vi "AnimatorFacade.vi"(0 "Data In":T6, 2 "Display State In":T2, 3 "Container State":T5) -> (6 "Data Out":T6, 7 "Display State Out":T2, 8 "Action":T1)   [LabVIEW 2019, in "AnimatorXControl.xctl"]
uses:
  AnimatorXControl.xctl
  AnimatorData.ctl
  <vilib>/_xctls/Container State.ctl
  AnimatorState.ctl
  <vilib>/picture/picture.llb/imagedata.ctl
  AnimatorSettings.ctl
  <vilib>/_xctls/Action.ctl
  AnimatorCommand.ctl
  <vilib>/_xctls/XControlSupport.lvlib
panel:
  out "Picture":picture
types:
  T1 = typedef "XControlSupport.lvlib/Action.ctl" = cluster{"Data Changed?":bool, "State Changed?":bool, "Action Name":string}
  T2 = typedef "AnimatorXControl.xctl/AnimatorState.ctl" = cluster{"Images":cluster{"Files":path[], "ImageData":T3[]}, "Settings":T4}
  T3 = typedef "imagedata.ctl" = cluster{"image type":i32, "image depth":i32, "image":u8[], "mask":u8[], "colors":u32[], "Rectangle":cluster{"left":i16, "top":i16, "right":i16, "bottom":i16}}
  T4 = typedef "AnimatorXControl.xctl/AnimatorSettings.ctl" = cluster{"Reverse":bool, "FrameRate":dbl, "WorkMode":enum16{"Automatic", "UseValue"}}
  T5 = typedef "XControlSupport.lvlib/Container State.ctl" = cluster{"Indicator?":bool, "Run Mode?":bool, " Refnum":refnum<vi>}
  T6 = typedef "AnimatorXControl.xctl/AnimatorData.ctl" = u32
  T7 = typedef "AnimatorXControl.xctl/AnimatorCommand.ctl" = enum16{"AddAnimator", "RemoveAnimator", "Settings"}
  T8 = cluster{"ImageData":picture[], "Pict Refnum":refnum<vi>}
  T9 = typedef "LVRectTypeDef.ctl" = cluster{"Left":i16, "Top":i16, "Right":i16, "Bottom":i16}
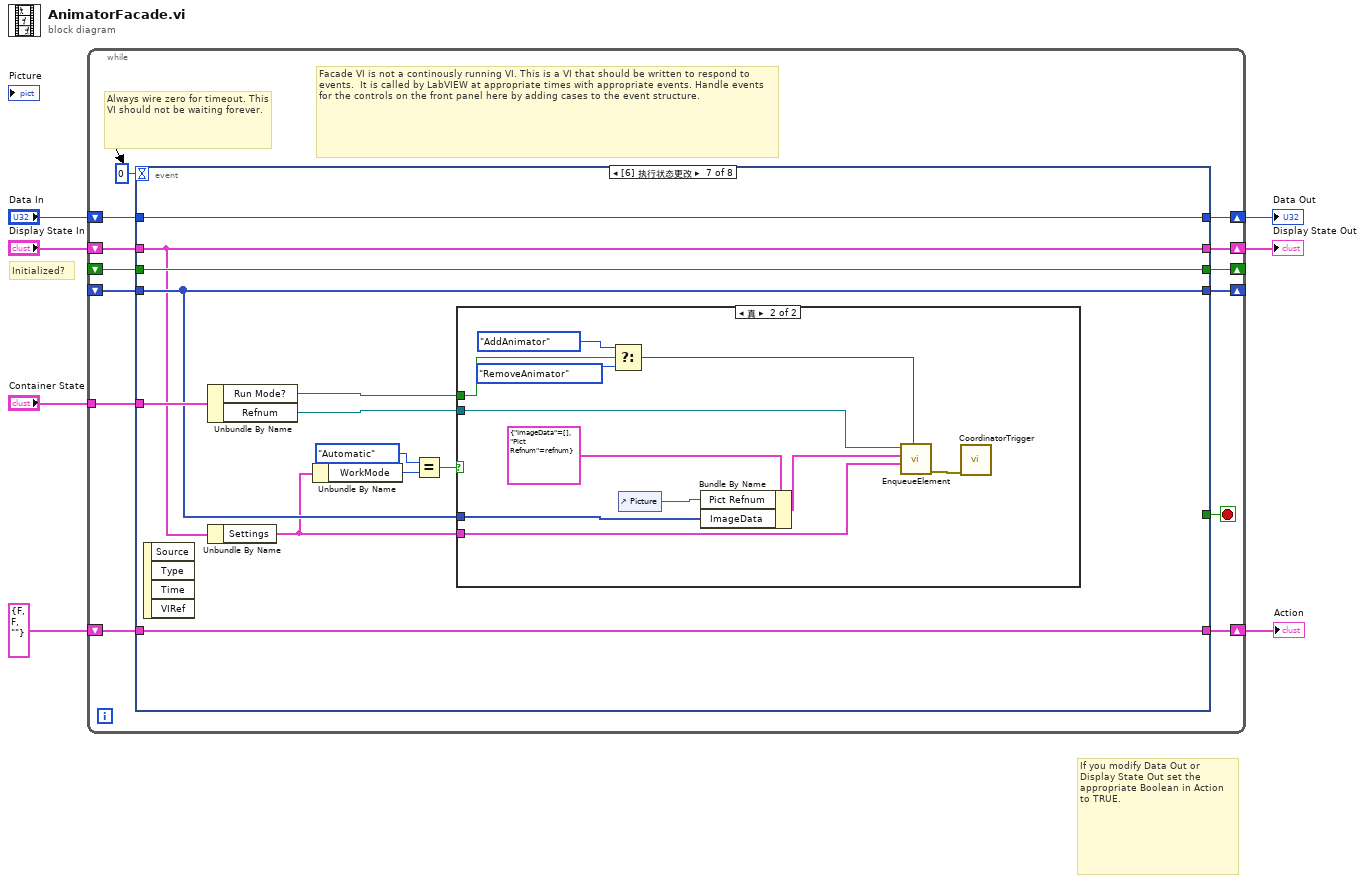
[diagram p0: block diagram]
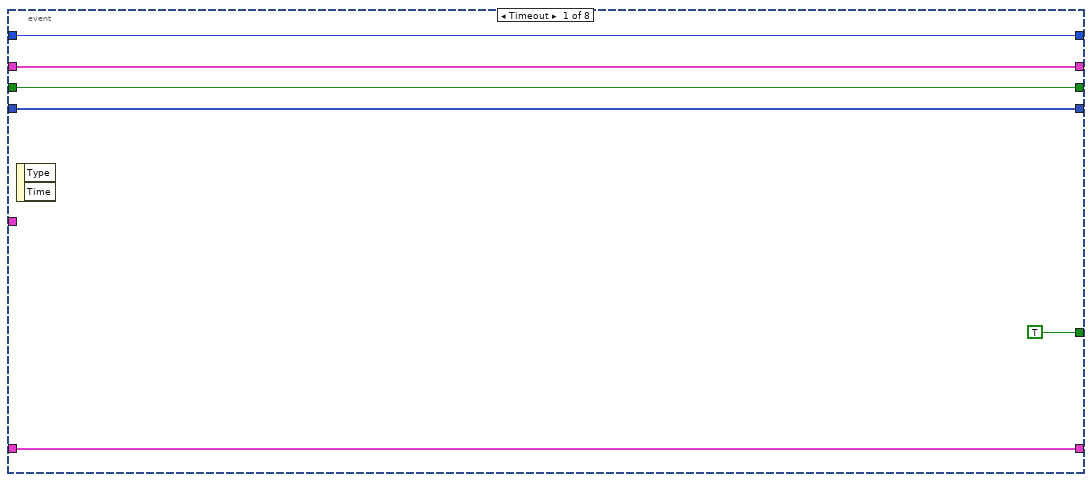
[diagram p2: hidden frame]
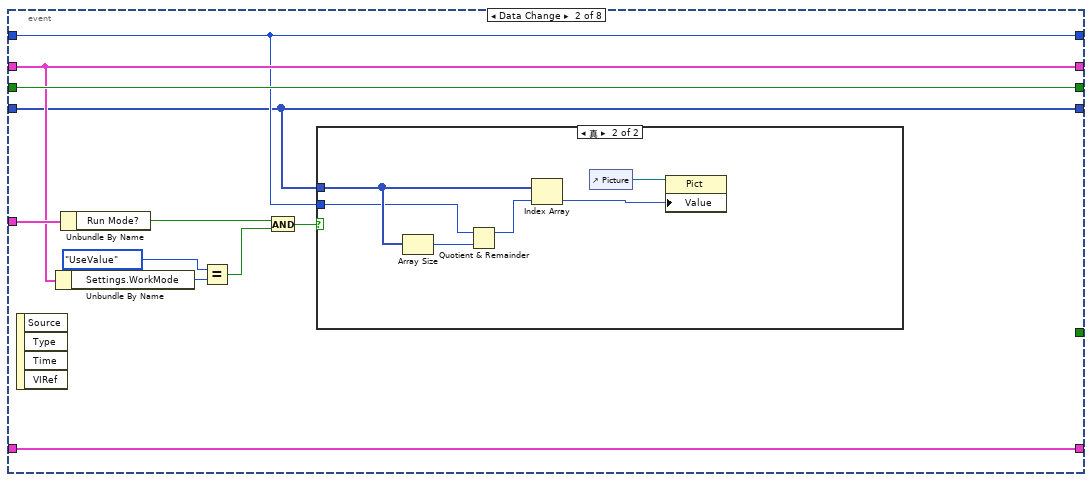
[diagram p3: hidden frame]
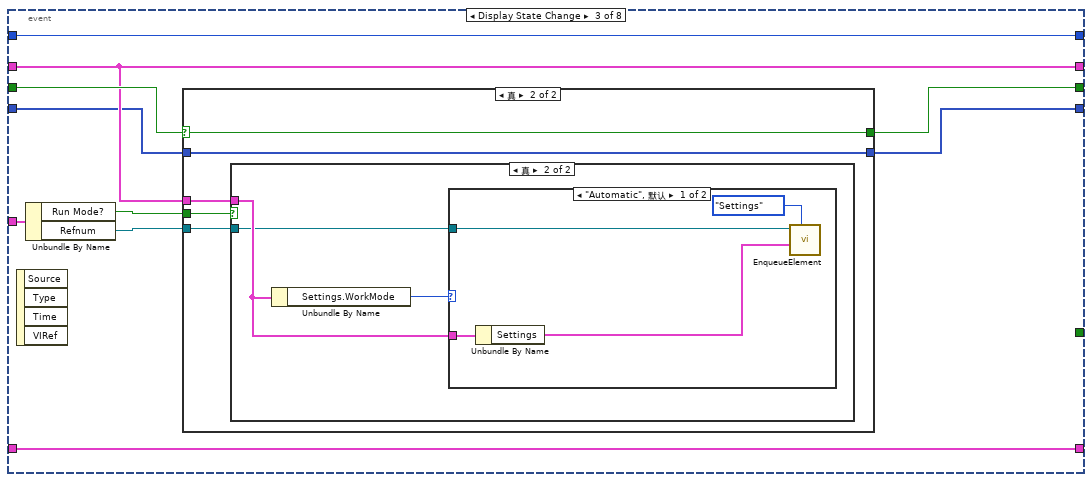
[diagram p5: hidden frame]
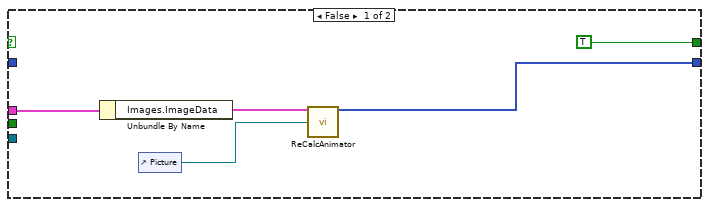
[diagram p6: hidden frame]
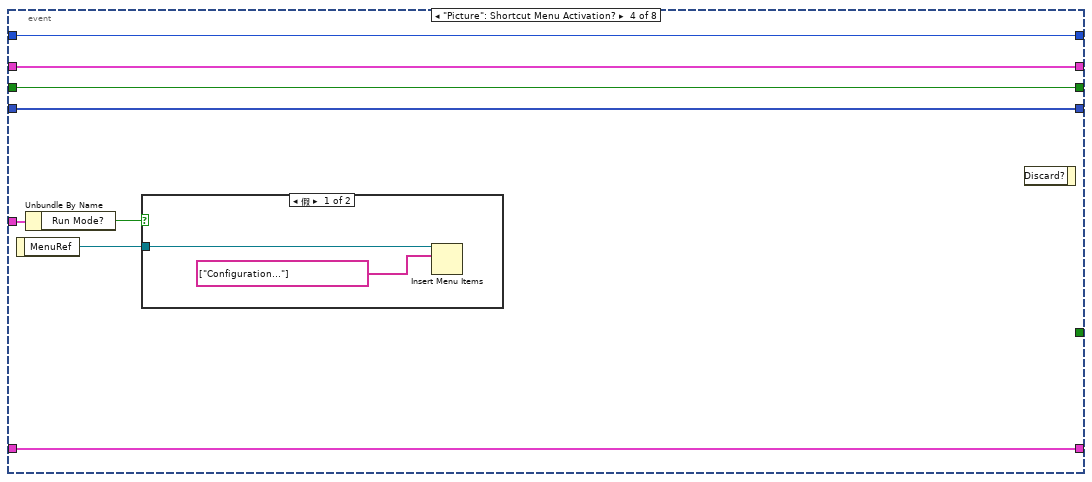
[diagram p9: hidden frame]
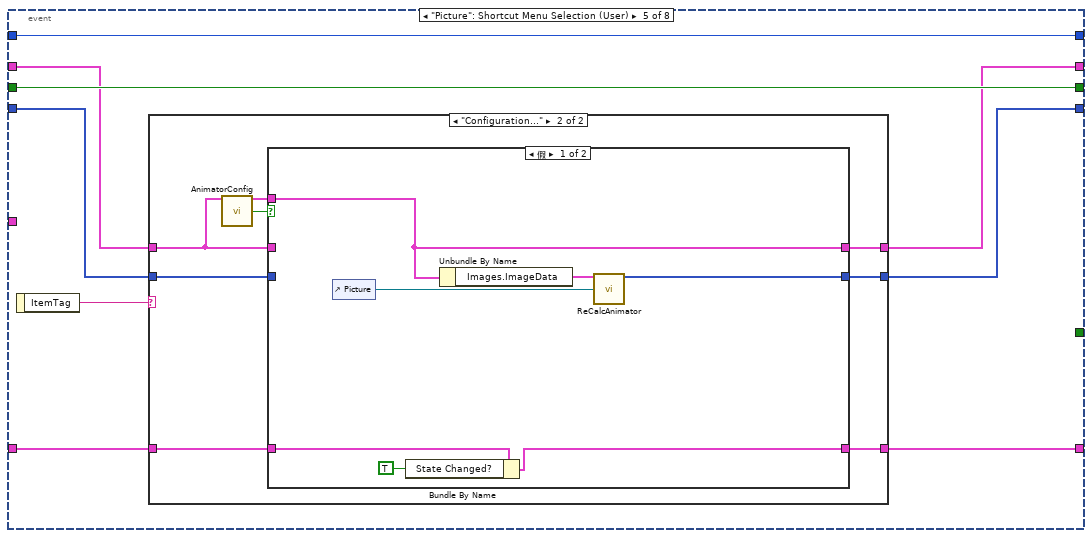
[diagram p11: hidden frame]
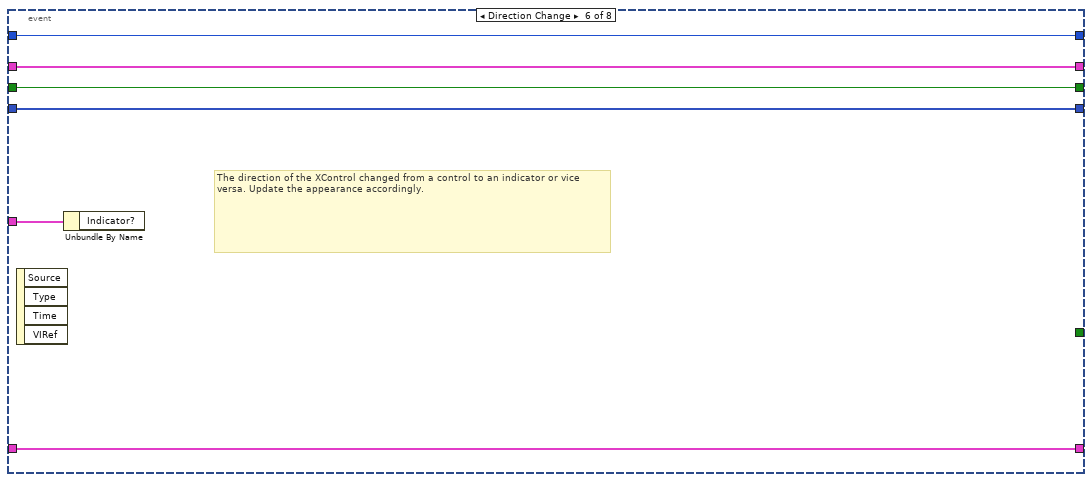
[diagram p14: hidden frame]
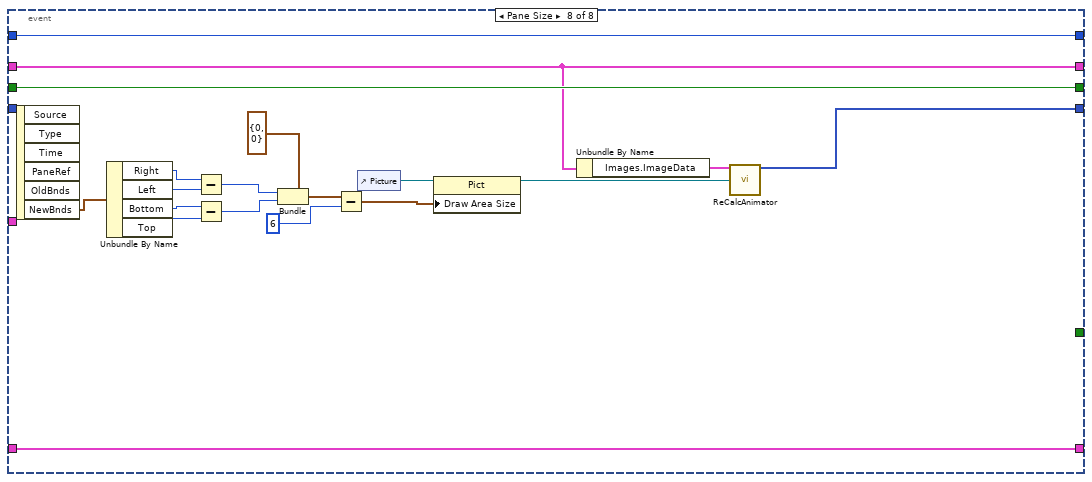
[diagram p16: hidden frame]
diagram:
  # "Initialized?"
  # "If you modify Data Out or\nDisplay State Out set the\nappropriate Boolean in Action\nto TRUE."
  n1 = while {
    shift-right: [w19] -> w4
    shift-left: "Display State In" -> [w20]
    tunnel: "Container State" -> [w16]
    shift-right: [w14] -> w7
    shift-left: "Data In" -> [w15]
    shift-right: [w12] -> w2
    shift-left: T1 {"Data Changed?"=FALSE, "State Changed?"=FALSE, "Action Name"=""} ("Action") -> [w13]
    shift-right: [w11] -> _
    shift-left: _ -> [w10]
    shift-right: [w8] -> _
    shift-left: _ -> [w9]
    stop <- w18 stop-if-true
    # "Facade VI is not a continously running VI. This is a VI that should be written to respond to events.  It is called by LabVIEW at appropriate times with appropriate events. Handle events for the controls on the front panel here by adding cases to the event structure."
    # "Always wire zero for timeout. This\nVI should not be waiting forever."
    n2 = event shown="[6] 执行状态更改" {
      selector: _ -> [_ _ _ _ _ _ _ _]
      dyn-events: _ -> [_ _ _ _ _ _ _ _]
      timeout: 0 -> [_ _ _ _ _ _ _ _]
      tunnel: w20 -> [w25 w34 w46 w74 w86 w115 w123 w144]
      tunnel: [w25 w34 w46 w74 w83 w115 w123 w144] -> w19
      tunnel: [TRUE _ _ _ _ _ _ _] -> w18
      tunnel: w16 -> [_ w35 w51 w78 _ w116 w128 _]
      tunnel: w15 -> [w24 w30 w53 w73 w89 w114 w127 w148]
      tunnel: [w24 w30 w53 w73 w89 w114 w127 w148] -> w14
      tunnel: [w26 w37 w47 w75 w84 w113 w126 w146] -> w12
      tunnel: w13 -> [w26 w37 w47 w75 w85 w113 w126 w146]
      tunnel: [w23 w36 w50 w72 w88 w112 w125 w147] -> w11
      tunnel: w10 -> [w23 w36 w52 w72 w88 w112 w125 w147]
      tunnel: w9 -> [w21 w29 w45 w71 w82 w111 w124 _]
      tunnel: [w21 w29 w44 w71 w81 w111 w124 w140] -> w8
      event Timeout {
        n3 = event-data() -> ()  [unwired: 1 in, 2 out]
      }
      event Data Change {
        n4 = event-data() -> ()  [unwired: 1 in, 4 out]
        n5 = Unbundle By Name(w34) -> ("Settings.WorkMode"=w32:enum16{"Automatic", "UseValue"})
        n6 = Unbundle By Name(w35) -> ("Run Mode?"=w28:bool)
        n7 = Equal?(x=enum16{"Automatic", "UseValue"}."UseValue", y=w32) -> (x = y?=w27:bool)
        n8 = And(x=w28, y=w27) -> (x .and. y?=w33:bool)
        n9 = case shown="真" w33 {
          tunnel: w30 -> [_ w38]
          tunnel: w29 -> [_ w43]
          frame False {
          }
          frame True {
            n10 = Array Size(array=w43) -> (size(s)=w39:i32)
            n11 = Quotient & Remainder(x=w38, y=w39) -> (x-y*floor(x/y)=w42:T6)  [unwired: 1 out]
            n12 = Index Array(array=w43, index=w42) -> (element=w40:picture)
            n13 = control-ref of="Picture"() -> (w41:refnum<vi>)
            n14 = property class="Pict"(reference=w41, "Value"=w40) -> ()  [unwired: 1 in, 2 out]
          }
        }
      }
      event Display State Change {
        n15 = event-data() -> ()  [unwired: 1 in, 4 out]
        n16 = Unbundle By Name(w51) -> ("Run Mode?"=w49:bool, "Refnum"=w48:refnum<vi>)
        n17 = case shown="真" w52 {
          selector: w52 -> [_ w63]
          tunnel: [TRUE w63] -> w50
          tunnel: w46 -> [w57 w61]
          tunnel: w49 -> [_ w62]
          tunnel: w48 -> [_ w60]
          tunnel: w45 -> [_ w59]
          tunnel: [w54 w59] -> w44
          frame False {
            n18 = Unbundle By Name(w57) -> ("Images.ImageData"=w55:T3[])
            n19 = control-ref of="Picture"() -> (w56:refnum<vi>)
            n20 = call "ReCalcAnimator.vi"("Image Array"=w55, "Pict Refnum"=w56) -> ("Pic Array"=w54:picture[])  [unwired: 12 in, 1 out]
          }
          frame True {
            n21 = case shown="真" w62 {
              tunnel: w61 -> [_ w65]
              tunnel: w60 -> [_ w64]
              frame False {
              }
              frame True {
                n22 = Unbundle By Name(w65) -> ("Settings.WorkMode"=w66:enum16{"Automatic", "UseValue"})
                n23 = case shown="\"Automatic\", 默认" w66 {
                  tunnel: w65 -> [w70 _]
                  tunnel: w64 -> [w68 _]
                  frame "Automatic", Default {
                    n24 = Unbundle By Name(w70) -> ("Settings"=w69:T4)
                    n25 = call "EnqueueElement.vi"("Command"=AnimatorCommand."Settings", "Settings"=w69, "XRefnum"=w68) -> ()  [unwired: 8 in, 1 out]
                  }
                  frame "UseValue" {
                  }
                }
              }
            }
          }
        }
      }
      event "Picture": Shortcut Menu Activation? {
        n26 = event-data() -> ("MenuRef"=w76:refnum<k9>)  [unwired: 1 in]
        n27 = Unbundle By Name(w78) -> ("Run Mode?"=w77:bool)
        n28 = case shown="假" w77 {
          tunnel: w76 -> [w80 _]
          frame False {
            n29 = Insert Menu Items(8:string[] ["Configuration..."] ("item names"), 9:w80) -> ()  [unwired: 4 in, 3 out]
          }
          frame True {
          }
        }
        n30 = event-data() -> ()  [unwired: 2 in, 1 out]
      }
      event "Picture": Shortcut Menu Selection (User) {
        n31 = event-data() -> ("ItemTag"=w87:string)  [unwired: 1 in]
        n32 = case shown="\"Configuration...\"" w87 {
          tunnel: w86 -> [w91 w96]
          tunnel: w85 -> [w92 w100]
          tunnel: [w92 w99] -> w84
          tunnel: [w91 w97] -> w83
          tunnel: [w90 w94] -> w81
          tunnel: w82 -> [w90 w93]
          frame Default {
          }
          frame "Configuration..." {
            n33 = call "AnimatorConfig.vi"("State In"=w96) -> ("State Out"=w98:T2, "Cancel?"=w95:bool)  [unwired: 12 in, 1 out]
            n34 = case shown="假" w95 {
              tunnel: w100 -> [w107 w110]
              tunnel: [w105 w110] -> w99
              tunnel: w98 -> [w104 _]
              tunnel: [w104 w109] -> w97
              tunnel: w96 -> [_ w109]
              tunnel: [w101 w108] -> w94
              tunnel: w93 -> [_ w108]
              frame False {
                n35 = control-ref of="Picture"() -> (w102:refnum<vi>)
                n36 = Bundle By Name(cluster=w107, "State Changed?"=TRUE) -> (w105:T1)
                n37 = Unbundle By Name(w104) -> ("Images.ImageData"=w103:T3[])
                n38 = call "ReCalcAnimator.vi"("Image Array"=w103, "Pict Refnum"=w102) -> ("Pic Array"=w101:picture[])  [unwired: 12 in, 1 out]
              }
              frame True {
              }
            }
          }
        }
      }
      event Direction Change {
        # "The direction of the XControl changed from a control to an indicator or vice versa. Update the appearance accordingly."
        n39 = event-data() -> ()  [unwired: 1 in, 4 out]
        n40 = Unbundle By Name(w116) -> ()  [unwired: 1 out]
      }
      event Exec State Change {
        n41 = event-data() -> ()  [unwired: 1 in, 4 out]
        n42 = Unbundle By Name(w128) -> ("Run Mode?"=w118:bool, "Refnum"=w117:refnum<vi>)
        n43 = Unbundle By Name(w123) -> ("Settings"=w119:T4)
        n44 = Unbundle By Name(w119) -> ("WorkMode"=w122:enum16{"Automatic", "UseValue"})
        n45 = Equal?(x=enum16{"Automatic", "UseValue"}."Automatic" ("y"), y=w122) -> (x = y?=w120:bool)
        n46 = case shown="真" w120 {
          tunnel: w117 -> [_ w132]
          tunnel: w124 -> [_ w135]
          tunnel: w119 -> [_ w138]
          tunnel: w118 -> [_ w137]
          frame False {
          }
          frame True {
            n47 = Select(t=AnimatorCommand."AddAnimator" ("Command"), s=w137, f=AnimatorCommand."RemoveAnimator" ("Command")) -> (s? t:f=w129:T7)
            n48 = control-ref of="Picture"() -> (w134:refnum<vi>)
            n49 = Bundle By Name(cluster=T8 {"ImageData"=[], "Pict Refnum"=refnum} ("ImageInfo"), "Pict Refnum"=w134, "ImageData"=w135) -> (w133:T8)
            n50 = call "EnqueueElement.vi"("Command"=w129, "Settings"=w138, "ImageInfo"=w133, "XRefnum"=w132) -> ("error out"=w139:errorcluster)  [unwired: 7 in]
            n51 = call "CoordinatorTrigger.vi"("error in (no error)"=w139) -> ()  [unwired: 10 in, 1 out]
          }
        }
      }
      event Pane Size {
        n52 = event-data() -> ("NewBnds"=w149:T9)  [unwired: 1 in, 5 out]
        n53 = Unbundle By Name(w149) -> ("Right"=w158:i16, "Left"=w157:i16, "Bottom"=w156:i16, "Top"=w155:i16)
        n54 = Subtract(x=w158, y=w157) -> (x-y=w153:i16)
        n55 = Subtract(x=w156, y=w155) -> (x-y=w154:i16)
        n56 = Bundle(cluster=cluster{"Height":i32, "Width":i32} {"Height"=0, "Width"=0} ("Rect"), "Height"=w153, "Width"=w154) -> (w152:cluster{"Height":i32, "Width":i32})
        n57 = Subtract(x=w152, y=6) -> (x-y=w151:cluster{"Height":i32, "Width":i32})
        n58 = control-ref of="Picture"() -> (w143:refnum<vi>)
        n59 = property class="Pict"(reference=w143, "Draw Area Size"=w151) -> (reference out=w141:refnum<vi>)  [unwired: 1 in, 1 out]
        n60 = Unbundle By Name(w144) -> ("Images.ImageData"=w142:T3[])
        n61 = call "ReCalcAnimator.vi"("Image Array"=w142, "Pict Refnum"=w141) -> ("Pic Array"=w140:picture[])  [unwired: 12 in, 1 out]
      }
    }
  }
  "Display State Out" <- w4
  "Data Out" <- w7
  "Action" <- w2
